vi "configuration.vi"(4 "force_read?":bool, 6 "config_file":path, 7 "command":T1=enum."read_config", 8 "error in (no error)":errorcluster, 11 "config in":T2) -> (0 "error out":errorcluster, 3 "config out":T2)   [LabVIEW 2015, in "lv-builder.lvlib"]
doc: "This VI is able to read/write configuration from all the associated modules defined in the master data cluster. It also acts as a functional global/data store in the event that no data has changed since the last write. It will self-initialize and well set an internal flag in the event an error is encountered when reading. If no command is provided, it will default to the read command."
uses:
  lv-builder.lvlib
  public/_controls/configuration.ctl
  _controls/command_configuration.ctl
  lv-build/lv-build.lvlib
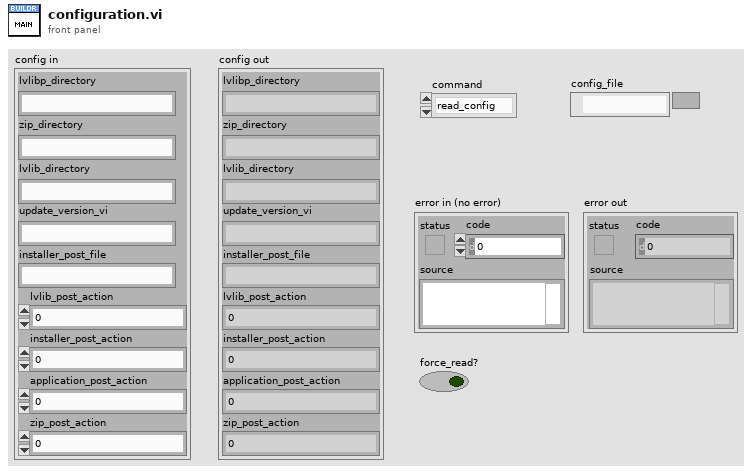
[diagram p1: front panel]
types:
  T1 = typedef "lv-builder.lvlib/command_configuration.ctl" = enum16{"<config_command>", "read_config", "write_config", "<null>"}
  T2 = typedef "lv-builder.lvlib/configuration.ctl" = cluster{"lvlibp_directory":string, "zip_directory":string, "lvlib_directory":string, "update_version_vi":string, "installer_post_file":string, "lvlib_post_action":u16, "installer_post_action":u16, "application_post_action":u16, "zip_post_action":u16}
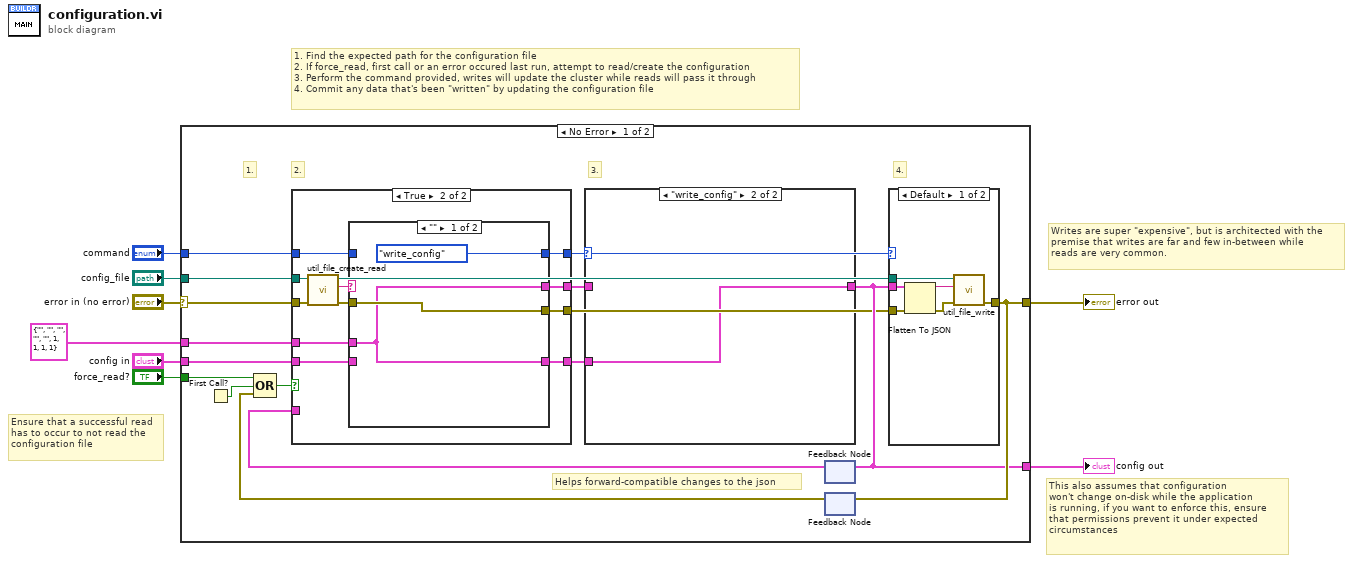
[diagram p0: block diagram]
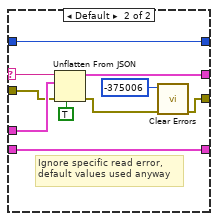
[diagram p3: hidden frame]
diagram:
  # "This also assumes that configuration\nwon't change on-disk while the application\nis running, if you want to enforce this, ensure\nthat permissions prevent it under expected\ncircumstances"
  # "1. Find the expected path for the configuration file\n2. If force_read, first call or an error occured last run, attempt to read/create the configuration\n3. Perform the command provided, writes will update the cluster while reads will pass it through\n4. Commit any data that's been \"written\" by updating the configuration file"
  # "Writes are super \"expensive\", but is architected with the\npremise that writes are far and few in-between while\nreads are very common."
  # "Ensure that a successful read\nhas to occur to not read the\nconfiguration file"
  n1 = case shown="No Error" "error in (no error)" {
    selector: "error in (no error)" -> [w10 w62]
    tunnel: "command" -> [w15 _]
    tunnel: [w24 w62] -> w4
    tunnel: "config in" -> [w13 _]
    tunnel: "config_file" -> [w9 _]
    tunnel: [w17 _] -> w3
    tunnel: "force_read?" -> [w21 _]
    tunnel: T2 {"lvlibp_directory"="", "zip_directory"="", "lvlib_directory"="", "update_version_vi"="", "installer_post_file"="", "lvlib_post_action"=1, "installer_post_action"=1, "application_post_action"=1, "zip_post_action"=1} ("default") -> [w18 _]
    frame No Error {
      # "Helps forward-compatible changes to the json"
      # "4."
      # "3."
      # "2."
      # "1."
      n2 = First Call?() -> (First Call?: T/F=w22:bool)
      n3 = feedback #1() -> (w19:T2)  [unwired: 1 in]
      n4 = feedback #2() -> (w23:errorcluster)  [unwired: 1 in]
      n5 = Compound Arithmetic op=OR(w21, w22, w23) -> (w20:bool)
      n6 = case shown="True" w20 {
        tunnel: w19 -> [w28 _]
        tunnel: w10 -> [w27 w37]
        tunnel: w9 -> [_ w38]
        tunnel: [w27 w35] -> w16
        tunnel: w18 -> [_ w39]
        tunnel: w15 -> [w26 w34]
        tunnel: [w26 w33] -> w14
        tunnel: w13 -> [w25 w32]
        tunnel: [w25 w31] -> w12
        tunnel: [w28 w30] -> w11
        frame False {
        }
        frame True {
          n7 = call "util_file_create_read.vi"("error in (no error)"=w37, "config_path"=w38) -> ("error out"=w36:errorcluster, "string"=w29:string)  [unwired: 8 in]
          n8 = case shown="\"\"" w29 {
            selector: w29 -> [_ w49]
            tunnel: w39 -> [w41 w52]
            tunnel: [w41 w51] -> w30
            tunnel: w36 -> [w42 w50]
            tunnel: [w42 w43] -> w35
            tunnel: w34 -> [_ w48]
            tunnel: [command_configuration."write_config" ("command") w48] -> w33
            tunnel: w32 -> [_ w47]
            tunnel: [w41 w47] -> w31
            frame "" {
            }
            frame Default {
              # "Ignore specific read error, \ndefault values used anyway"
              n9 = Unflatten From JSON(JSON string=w49, type and defaults=w52, default null elements? (F)=TRUE, error in (no error)=w50) -> (value=w51:T2, error out=w45:errorcluster)  [unwired: 3 in]
              n10 = call <vilib>:"Clear Errors.vi"("error in (no error)"=w45, "specific error code to clear (0: all)"=-375006) -> ("error out"=w43:errorcluster)  [unwired: 4 in, 1 out]
            }
          }
        }
      }
      n11 = case shown="\"write_config\"" w14 {
        tunnel: w12 -> [_ w61]
        tunnel: [w60 w61] -> w17
        tunnel: w11 -> [w60 _]
        frame Default {
        }
        frame "write_config" {
        }
      }
      n12 = feedback-in #1(w17) -> ()
      n13 = case shown="Default" w14 {
        tunnel: w17 -> [w55 _]
        tunnel: w16 -> [w56 w59]
        tunnel: [w53 w59] -> w24
        tunnel: w9 -> [w54 _]
        frame Default {
          n14 = Flatten To JSON(anything=w55, error in (no error)=w56) -> (JSON string=w58:string, 11:w57:errorcluster)  [unwired: 1 in]
          n15 = call "util_file_write.vi"("error in (no error)"=w57, "string"=w58, "config_path"=w54) -> ("error out"=w53:errorcluster)  [unwired: 8 in]
        }
        frame "<config_command>", "read_config", "<null>" {
        }
      }
      n16 = feedback-in #2(w24) -> ()
    }
    frame Error {
      # "If an error is wired in, be sure to skip over functionality to preserve the original error"
    }
  }
  "config out" <- w3
  "error out" <- w4
